vi "Move to possition.vi"(8 "error in (no error)":errorcluster, 10 "absolute possition(rev)":dbl, 11 "Motor in":refnum<class "Motor.lvclass">) -> (0 "error out":errorcluster, 3 "Motor out":refnum<class "Motor.lvclass">)   [LabVIEW 2019, in "Motor.lvclass"]
uses:
  Motor.lvclass
  Motor.lvclass/Motor.ctl
  Motor Serial class/Serial.lvclass
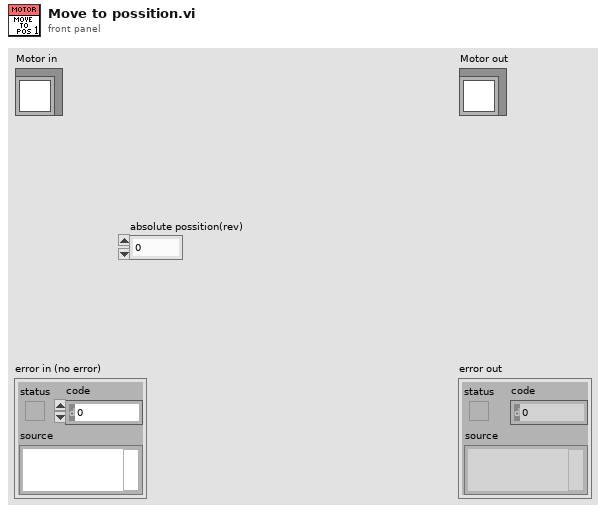
[diagram p1: front panel]
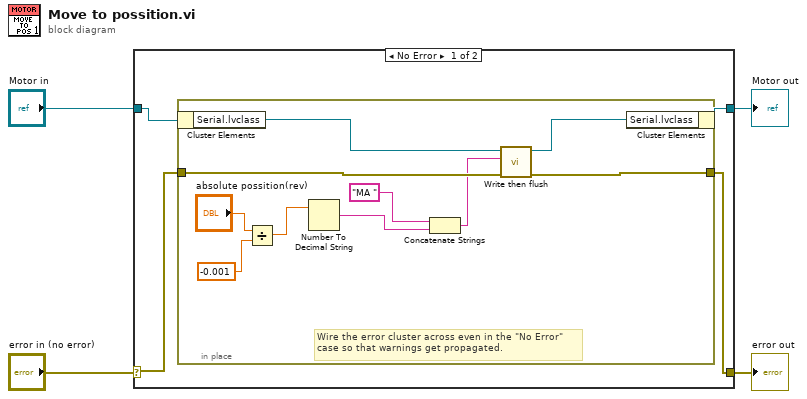
[diagram p0: block diagram]
diagram:
  n1 = case shown="No Error" "error in (no error)" {
    selector: "error in (no error)" -> [w6 w20]
    tunnel: [w5 w20] -> w3
    tunnel: [w7 w19] -> w1
    tunnel: "Motor in" -> [w8 w19]
    frame No Error {
      n2 = in-place {
        in-place-border: w6 -> [w16]
        in-place-border: [w15] -> w5
        # "Wire the error cluster across even in the \"No Error\"\ncase so that warnings get propagated."
        n3 = in-place-cluster #1(w8) -> ("Serial.lvclass"=w18:refnum<class "Serial.lvclass">)
        n4 = Divide(x="absolute possition(rev)", y=-0.001) -> (x/y=w12:dbl)
        n5 = Number To Decimal String(number=w12) -> (decimal integer string=w10:string)  [unwired: 1 in]
        n6 = Concatenate Strings("MA " ("string"), w10) -> (w9:string)
        n7 = call "Write then flush.vi"("error in (no error)"=w16, "TX Data"=w9, "Motor_Serial in"=w18) -> ("error out"=w15:errorcluster, "Motor_Serial out"=w17:refnum<class "Serial.lvclass">)  [unwired: 7 in]
        n8 = in-place-cluster #1("Serial.lvclass"=w17) -> (w7:refnum<class "Motor.lvclass">)
      }
    }
    frame Error {
    }
  }
  "error out" <- w3
  "Motor out" <- w1
